vi "response_total_bytes.vi"(8 "error in (no error)":errorcluster, 11 "Request in":refnum<class "Request.lvclass">) -> (0 "error out":errorcluster, 2 "total_bytes":u64, 3 "Request out":refnum<class "Request.lvclass">)   [LabVIEW 2020, in "reqwest.lvlib" / "Request.lvclass"]
uses:
  Request/Request.lvclass
  Request/Request.lvclass/Request.ctl
  lv_reqwest_64.dll
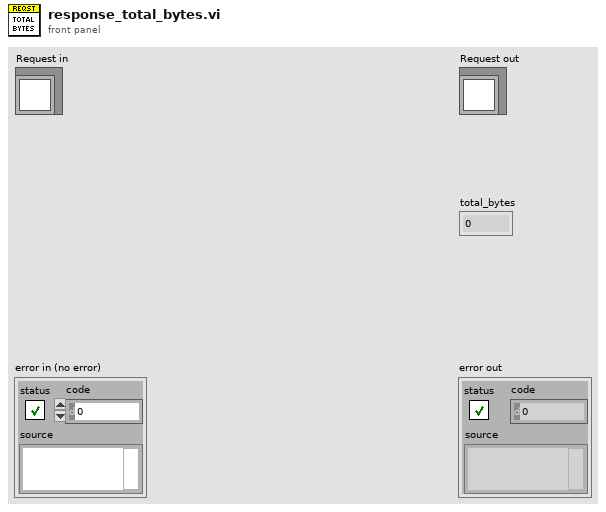
[diagram p1: front panel]
types:
  T1 = typedef "reqwest.lvlib/Request.lvclass/request_id_int.ctl" = i32
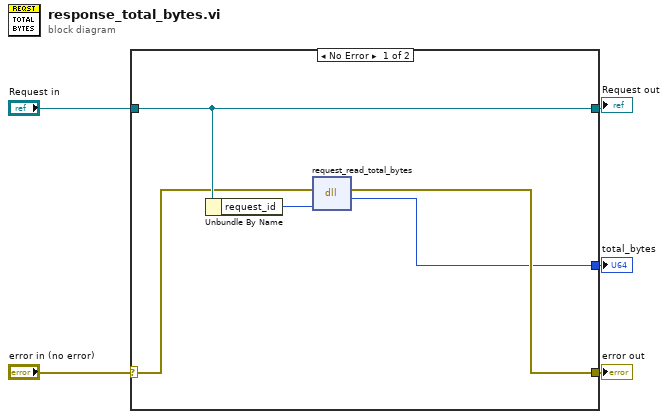
[diagram p0: block diagram]
diagram:
  n1 = case shown="No Error" "error in (no error)" {
    selector: "error in (no error)" -> [w8 w11]
    tunnel: "Request in" -> [w9 w12]
    tunnel: [w6 _] -> w3
    tunnel: [w10 w11] -> w1
    tunnel: [w9 w12] -> w2
    frame No Error {
      n2 = Unbundle By Name(w9) -> ("request_id"=w7:T1)
      n3 = dll-call lib="C:/Projects/reqwest-rs-labview/lv_src/lv_reqwest_64.dll" fn="request_read_total_bytes"(error in=w8, "request_id"=w7) -> (error out=w10:errorcluster, "total_bytes"=w6:u64)  [unwired: 3 in, 1 out]
    }
    frame Error {
    }
  }
  "error out" <- w1
  "total_bytes" <- w3
  "Request out" <- w2
